vi "NyquistTrimCoefficients.vi"(7 "Cutoff type":string(combo), 9 "InterpolatedCoefficients":dbl[](array[numeric]), 10 "Frequencies":dbl[](array[numeric]), 11 "fs (Hz)":dbl) -> (1 "NyquistLimitedCoefficients":dbl[](array[numeric]), 3 "NyquistFreq":dbl)   [LabVIEW 2011]
uses:
  <vilib>/Analysis/NI_AALBase.lvlib
panel:
  in  "cosineFadeLength":i32=12
  out "XY Graph":cluster{"Frequencies":dbl[], dbl[]}[](graph)
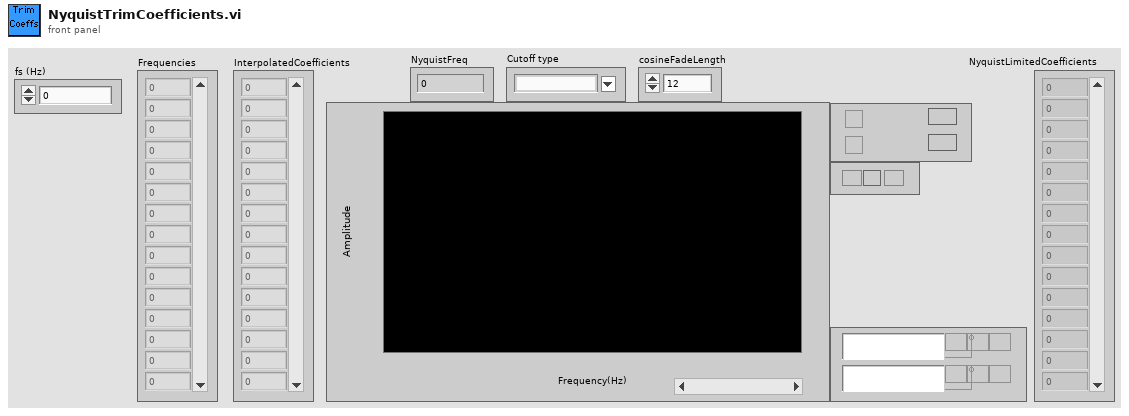
[diagram p1: front panel]
types:
  T1 = cluster{"Frequencies":dbl[], "InterpolatedCoefficients":dbl[]}
  T2 = cluster{"Frequencies":dbl[], "InterpolatedCoefficients":dbl[]}[]
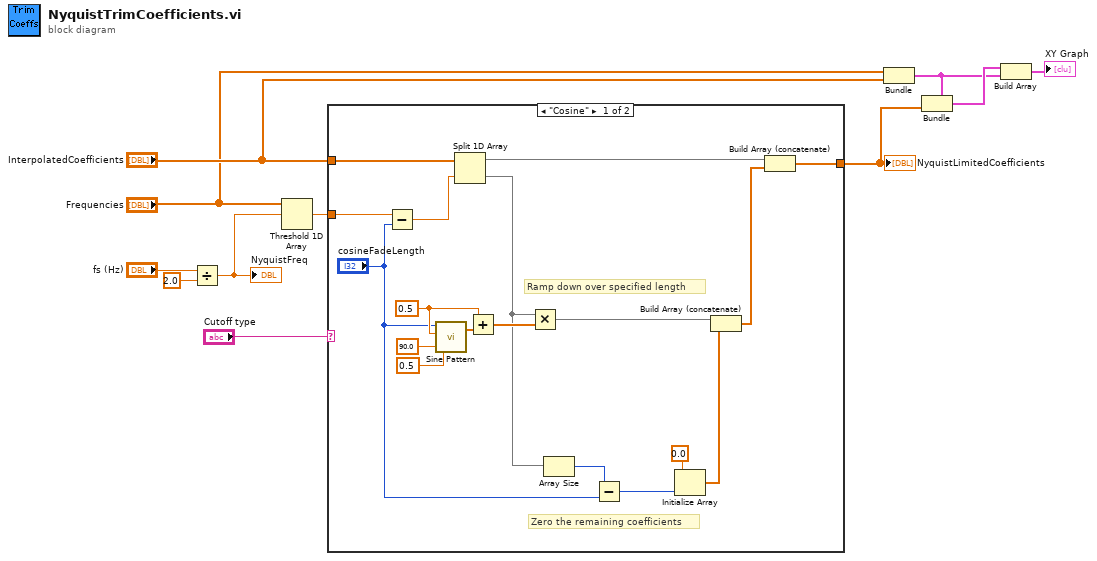
[diagram p0: block diagram]
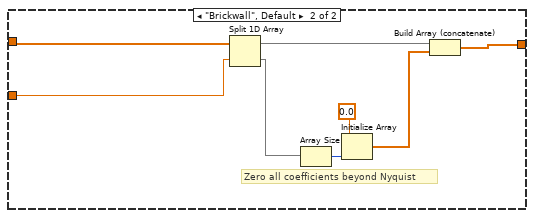
[diagram p2: hidden frame]
diagram:
  n1 = Divide(x="fs (Hz)", y=2.0) -> (x/y=w8:dbl)
  "NyquistFreq" <- w8
  n2 = Threshold 1D Array(2:w8, 3:"Frequencies") -> (0:w7:dbl)  [unwired: 1 in]
  n3 = case shown="\"Cosine\"" "Cutoff type" {
    tunnel: "InterpolatedCoefficients" -> [w19 w35]
    tunnel: [w18 w31] -> w6
    tunnel: w7 -> [w17 w30]
    frame "Cosine" {
      w26 = 0.5 ("amplitude")
      # "Ramp down over specified length"
      # "Zero the remaining coefficients"
      n4 = Subtract(x=w17, y="cosineFadeLength") -> (x-y=w16:dbl)
      n5 = call <vilib>:"Sine Pattern.vi"("cycles"=0.5, "phase(degrees)"=90.0, "amplitude"=w26, "samples"="cosineFadeLength") -> ("Sinusoidal Pattern"=w28:dbl[])  [unwired: 1 out]
      n6 = Split 1D Array(array=w19, index=w16) -> (first subarray=w20:dbl[], second subarray=w12:dbl[])
      n7 = Add(x=w26, y=w28) -> (x+y=w15:dbl[])
      n8 = Multiply(x=w12, y=w15) -> (x*y=w24:dbl[])
      n9 = Array Size(array=w12) -> (size(s)=w23:i32)
      n10 = Subtract(x=w23, y="cosineFadeLength") -> (x-y=w22:i32)
      n11 = Initialize Array(0.0 ("element"), w22) -> (w21:dbl[])
      n12 = Build Array (concatenate)(w24, w21) -> (w14:dbl[])
      n13 = Build Array (concatenate)(w20, w14) -> (w18:dbl[])
    }
    frame "Brickwall", Default {
      # "Zero all coefficients beyond Nyquist"
      n14 = Split 1D Array(array=w35, index=w30) -> (first subarray=w32:dbl[], second subarray=w34:dbl[])
      n15 = Array Size(array=w34) -> (size(s)=w37:i32)
      n16 = Initialize Array(0.0 ("element"), w37) -> (w33:dbl[])
      n17 = Build Array (concatenate)(w32, w33) -> (w31:dbl[])
    }
  }
  "NyquistLimitedCoefficients" <- w6
  n18 = Bundle("Frequencies"="Frequencies", "InterpolatedCoefficients"="InterpolatedCoefficients") -> (w1:T1)  [unwired: 1 in]
  n19 = Bundle(cluster=w1, "InterpolatedCoefficients"=w6) -> (w2:T1)  [unwired: 1 in]
  n20 = Build Array(w2, w1) -> (→"XY Graph":T2)
